vi "stop.vi"(8 "error in (no error)":errorcluster, 10 "stop?":bool, 11 "HWController in":refnum<class "HWController.lvclass">) -> (0 "error out":errorcluster, 2 "stopped":bool, 3 "HWController out":refnum<class "HWController.lvclass">)   [LabVIEW 2011, in "Hardware.lvlib" / "HWControllers.lvlib" / "HWController.lvclass"]
uses:
  HWController.lvclass
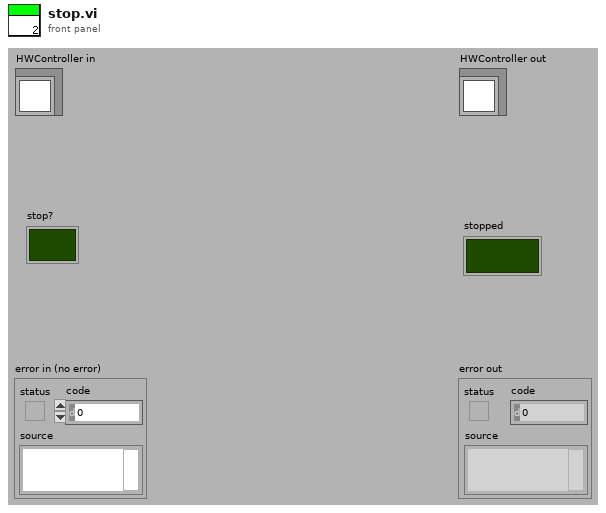
[diagram p1: front panel]
types:
  T1 = enum16{"Ready", "Compiling", "Configured", "Running", "Stopping", "Unresolved Error"}
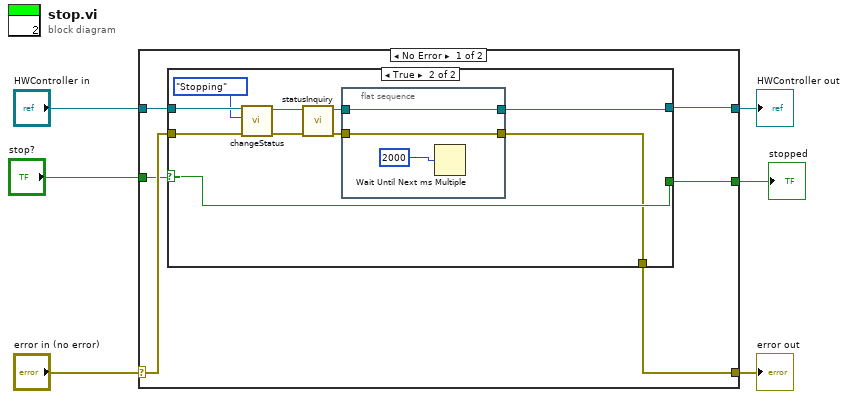
[diagram p0: block diagram]
diagram:
  n1 = case shown="No Error" "error in (no error)" {
    selector: "error in (no error)" -> [w11 w31]
    tunnel: [w9 w31] -> w5
    tunnel: [w10 w30] -> w4
    tunnel: "HWController in" -> [w12 w30]
    tunnel: "stop?" -> [w8 w29]
    tunnel: [w7 w29] -> w1
    frame No Error {
      n2 = case shown="True" w8 {
        selector: w8 -> [w15 w21]
        tunnel: w12 -> [w14 w23]
        tunnel: w11 -> [w13 w22]
        tunnel: [w14 w18] -> w10
        tunnel: [w13 w17] -> w9
        tunnel: [w15 w21] -> w7
        frame False {
        }
        frame True {
          n3 = call "changeStatus.vi"("error in (no error)"=w22, "status"=T1."Stopping", "HWController in"=w23) -> ("error out"=w25:errorcluster, "HWController out"=w24:refnum<class "HWController.lvclass">)  [unwired: 7 in]
          n4 = call-dynamic "statusInquiry.vi"("error in (no error)"=w25, "HWController in"=w24) -> ("error out"=w19:errorcluster, "HWController out"=w20:refnum<class "HWController.lvclass">)  [unwired: 8 in]
          n5 = flat-sequence {
            tunnel: w20 -> [w28]
            tunnel: w19 -> [w27]
            tunnel: [w28] -> w18
            tunnel: [w27] -> w17
            frame #0 {
              n6 = Wait Until Next ms Multiple(millisecond multiple=2000) -> ()  [unwired: 1 out]
            }
          }
        }
      }
    }
    frame Error {
    }
  }
  "error out" <- w5
  "HWController out" <- w4
  "stopped" <- w1
